vi "isAsserted.vi"(11 "Leaf.Assertion":refnum<class "Leaf.Assertion.lvclass">) -> (1 "UpstreamError":bool, 2 "Asserted":bool, 3 "Leaf.Assertion":refnum<class "Leaf.Assertion.lvclass">)   [LabVIEW 2021, in "Bananas.lvlib" / "Leaf.Assertion.lvclass"]
uses:
  Leaf.Assertion.lvclass
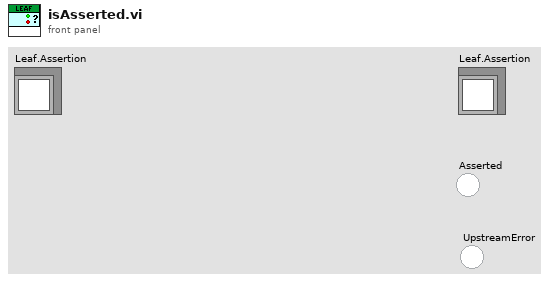
[diagram p1: front panel]
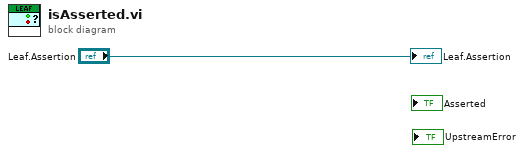
[diagram p0: block diagram]
diagram:
  "Leaf.Assertion" <- "Leaf.Assertion"
